vi "RichToFlatcif_plugincore_GetVersionResponse.vi"(5 "OutputClusterType":T1, 11 "InputCluster":T3) -> (3 "OutputCluster":T1)   [LabVIEW 2021, in "CIFCorePlugin_server.lvlib"]
uses:
  CIFCorePlugin_server.lvlib
  cif_plugincore_GetVersionResponse.ctl
  cif_common_Version.ctl
  cif_plugincore_GetVersionResponse_Flat.ctl
  cif_common_Version_Flat.ctl
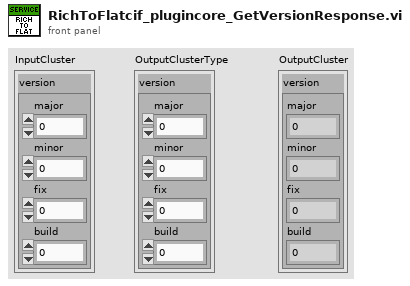
[diagram p1: front panel]
types:
  T1 = typedef "CIFCorePlugin_server.lvlib/cif_plugincore_GetVersionResponse_Flat.ctl" = cluster{"version":T2}
  T2 = typedef "CIFCorePlugin_server.lvlib/cif_common_Version_Flat.ctl" = cluster{"major":u32, "minor":u32, "fix":u32, "build":u32}
  T3 = typedef "CIFCorePlugin_server.lvlib/cif_plugincore_GetVersionResponse.ctl" = cluster{"version":T4}
  T4 = typedef "CIFCorePlugin_server.lvlib/cif_common_Version.ctl" = cluster{"major":u32, "minor":u32, "fix":u32, "build":u32}
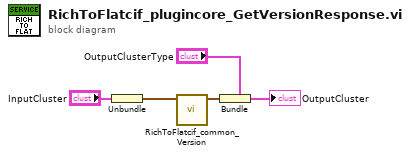
[diagram p0: block diagram]
diagram:
  n1 = Unbundle "Unbundle"("InputCluster") -> ("version"=w2:T4)
  n2 = call "RichToFlatcif_common_Version.vi"("InputCluster"=w2) -> ("OutputCluster"=w1:T2)  [unwired: 10 in]
  n3 = Bundle "Bundle"(cluster="OutputClusterType", "version"=w1) -> (→"OutputCluster":T1)
